vi "Keith 7001 Arm Lay 2 Config.vi"(1 "delay period (sec)":dbl min=0.0 max=99999.999 format="%.3f", 2 "timer interval (sec)":dbl=0.001 min=0.001 max=99999.999 format="%.3f", 3 "trigger link output":u16=2 min=1 max=6 step=1, 4 "trigger link input":u16=1 min=1 max=6 step=1, 5 "count value":u16=1 min=1 max=9999, 6 "count":bool=TRUE, 7 "error in":T1, 8 "source bypass":bool, 9 "source (immediate:1)":u16(ring)=1 items=["hold", "immediate", "timer", "manual", "GPIB", "trigger link", "external"], 10 "GPIB address":string="7") -> (0 "error out":T1)   [LabVIEW 2019]
doc: "This VI for the Keithley 7001 Switch System is used to configure the scan layer (arm layer 2)."
panel:
  # "set finite value\ninfinite"
  # "enable (source)\ndisable (acceptor)"
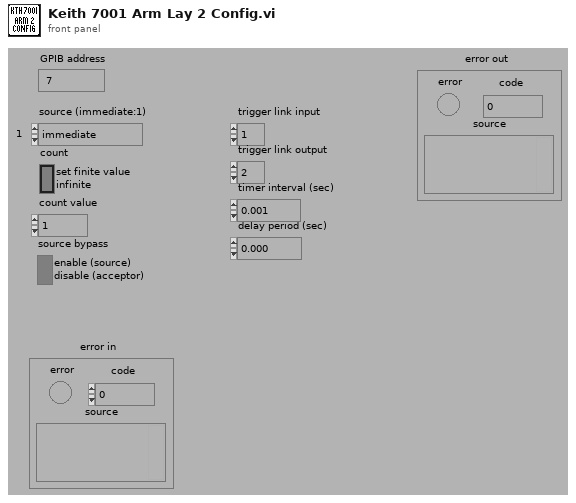
[diagram p1: front panel]
types:
  T1 = cluster{"error":bool, "code":i32, "source":string}
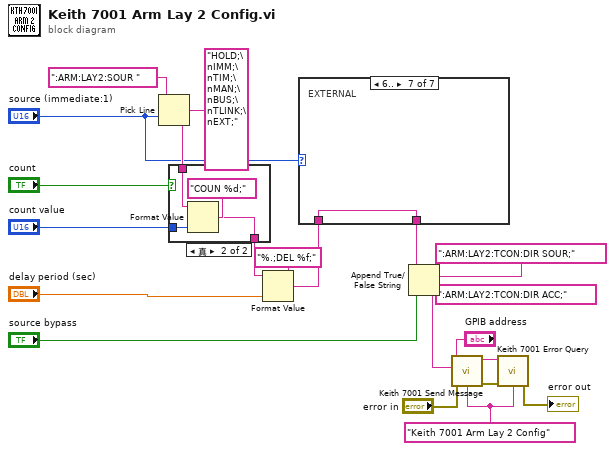
[diagram p0: block diagram]
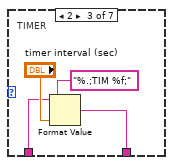
[diagram p4: hidden frame]
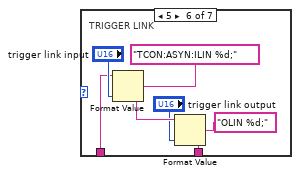
[diagram p7: hidden frame]
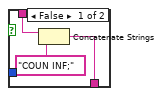
[diagram p8: hidden frame]
diagram:
  w1 = "Keith 7001 Arm Lay 2 Config"
  n1 = Pick Line(string ("")=":ARM:LAY2:SOUR ", multi-line string="HOLD;\nIMM;\nTIM;\nMAN;\nBUS;\nTLINK;\nEXT;", line index="source (immediate:1)") -> (output string=w19:string)
  n2 = case shown="真" "count" {
    tunnel: w19 -> [w24 w28]
    tunnel: [w22 w25] -> w17
    tunnel: "count value" -> [_ w27]
    frame False {
      n3 = Concatenate Strings(w24, "COUN INF;") -> (w22:string)
    }
    frame True {
      n4 = Format Value(string ("")=w28, format string="COUN %d;", value (0)=w27) -> (output string=w25:string)
    }
  }
  n5 = Format Value(string ("")=w17, format string="%.;DEL %f;", value (0)="delay period (sec)") -> (output string=w13:string)
  n6 = case shown="6.." "source (immediate:1)" {
    tunnel: w13 -> [w29 w30 w33 w35 w36 w41 w44]
    tunnel: [w29 w30 w31 w35 w36 w37 w44] -> w11
    frame ..0 {
      # "HOLD"
    }
    frame 1 {
      # "IMMEDIATE"
    }
    frame 2 {
      # "TIMER"
      n7 = Format Value(string ("")=w33, format string="%.;TIM %f;", value (0)="timer interval (sec)") -> (output string=w31:string)
    }
    frame 3 {
      # "MANUAL"
    }
    frame 4 {
      # "GPIB"
    }
    frame 5 {
      # "TRIGGER LINK"
      n8 = Format Value(string ("")=w41, format string="TCON:ASYN:ILIN %d;", value (0)="trigger link input") -> (output string=w40:string)
      n9 = Format Value(string ("")=w40, format string="OLIN %d;", value (0)="trigger link output") -> (output string=w37:string)
    }
    frame 6.. {
      # "EXTERNAL"
    }
  }
  n10 = Append True/False String(1:"source bypass", 2:":ARM:LAY2:TCON:DIR ACC;", 3:":ARM:LAY2:TCON:DIR SOUR;", 4:w11) -> (0:w8:string)
  n11 = call "Keith 7001 Send Message.vi"("address string"="GPIB address", "write buffer"=w8, "source"=w1, "error in"="error in") -> ("address out"=w2:string, "error out"=w3:T1)  [unwired: 2 in, 2 out]
  n12 = call "Keith 7001 Error Query.vi"("GPIB address"=w2, "error in"=w3, "source"=w1) -> ("error out"=→"error out":T1)  [unwired: 2 out]
